vi "Sound Generator Example.vi"() -> ()   [LabVIEW 2018]
uses:
  Waveform Control.xctl
  <vilib>/Waveform/WDTOps.llb/WDT Append Waveforms DBL.vi
panel:
  in  "Show Y=0":bool=TRUE
  in  "Show Scales":bool
  in  "Exit":bool
  in  "Secs to play":dbl=0.25
  in  "Repeats/sec":dbl=478.0
  in  "Play":bool
  in  "Waveform":waveform(dbl)(xcontrol)={"t0"=timestamp(0 s since 1904-01-01), "dt"=0.0, "Y"=[0.0, 0.049067674327418015, 0.0980171403295606, 0.14673047445536175, 0.19509032201612828, 0.2429801799032639, 0.2902846772544624, 0.33688985339222005, 0.3826834323650898, 0.4275550934302821, 0.47139673682599764, 0.5141027441932218, 0.5555702330196022, 0.5956993044924334, 0.6343932841636455, 0.6715589548470184, 0.7071067811865475, 0.7409511253549591, 0.7730104533627369, 0.8032075314806449, 0.8314696123025451, 0.8577286100002721, 0.8819212643483549, 0.9039892931234433, 0.9238795325112866, 0.9415440651830208, 0.9569403357322087, 0.970031253194544, 0.9807852804032303, 0.9891765099647809, 0.9951847266721968, 0.9987954562051723, 0.9999999999999999, 0.9987954562051723, 0.9951847266721968, 0.9891765099647809, 0.9807852804032304, 0.970031253194544, 0.9569403357322088, 0.9415440651830208, 0.9238795325112867, 0.9039892931234433, 0.881921264348355, 0.8577286100002721, 0.8314696123025452, 0.8032075314806449, 0.773010453362737, 0.7409511253549591, 0.7071067811865476, 0.6715589548470184, 0.6343932841636456, 0.5956993044924334, 0.5555702330196023, 0.5141027441932218, 0.4713967368259977, 0.42755509343028214, 0.38268343236508984, 0.3368898533922201, 0.29028467725446244, 0.24298017990326393, 0.19509032201612836, 0.14673047445536178, 0.0980171403295607, 0.04906767432741803, 1.0034968732711147e-16, -0.04906767432741801, -0.0980171403295605, -0.14673047445536175, -0.19509032201612816, -0.2429801799032639, -0.2902846772544623, -0.33688985339222005, -0.38268343236508967, -0.4275550934302821, -0.47139673682599753, -0.5141027441932218, -0.5555702330196021, -0.5956993044924334, -0.6343932841636454, -0.6715589548470184, -0.7071067811865475, -0.7409511253549591, -0.7730104533627369, -0.8032075314806449, -0.8314696123025451, -0.8577286100002721, -0.8819212643483549, -0.9039892931234433, -0.9238795325112866, -0.9415440651830208, -0.9569403357322087, -0.970031253194544, -0.9807852804032303, -0.9891765099647809, -0.9951847266721968, -0.9987954562051723, -0.9999999999999999, -0.9987954562051723, -0.9951847266721968, -0.9891765099647809, -0.9807852804032304, -0.970031253194544, -0.9569403357322088, -0.9415440651830208, -0.9238795325112867, -0.9039892931234433, -0.881921264348355, -0.8577286100002721, -0.8314696123025452, -0.8032075314806449, -0.773010453362737, -0.7409511253549591, -0.7071067811865476, -0.6715589548470184, -0.6343932841636456, -0.5956993044924334, -0.5555702330196023, -0.5141027441932218, -0.4713967368259977, -0.42755509343028214, -0.38268343236508984, -0.3368898533922201, -0.29028467725446244, -0.24298017990326395, -0.19509032201612836, -0.1467304744553618, -0.0980171403295607, -0.049067674327418064], "attributes"=variant("XControl State"=variant(cluster{"Show Axes":bool, "Show Y=0":bool, "Controls":cluster{"Type":enum16{"Level", "Sine", "Triangle", "Ramp", "Saw Tooth", "Square", "Function"}, "Periods":dbl, "Points":i32, "Offset":dbl, "Amplitdue":dbl, "Starting Phase":dbl, "func":string}, "Show Current Location":bool, "Current Location":i32, "dt":dbl, "t0":timestamp} {"Show Axes"=FALSE, "Show Y=0"=TRUE, "Controls"={"Type"=enum."Sine", "Periods"=1.0, "Points"=128, "Offset"=0.0, "Amplitdue"=1.0, "Starting Phase"=0.0, "func"=""}, "Show Current Location"=TRUE, "Current Location"=0, "dt"=0.0, "t0"=timestamp(0 s since 1904-01-01)}))}
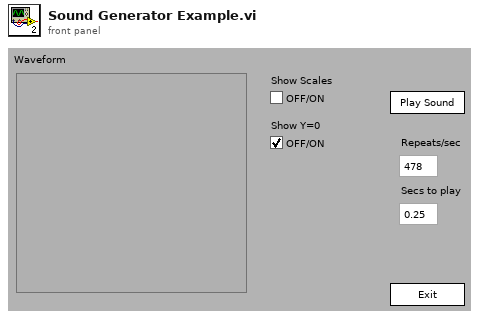
[diagram p1: front panel]
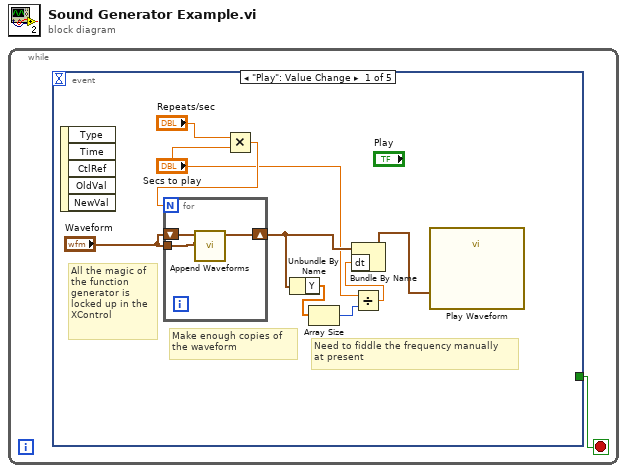
[diagram p0: block diagram]
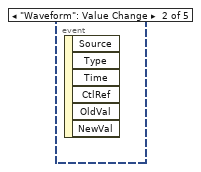
[diagram p2: hidden frame]
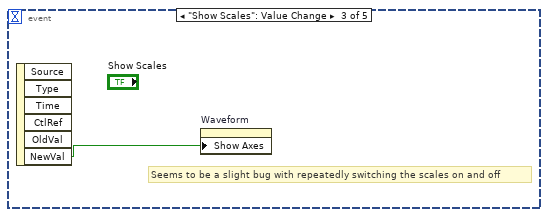
[diagram p3: hidden frame]
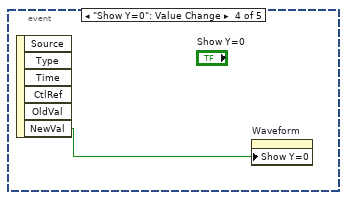
[diagram p4: hidden frame]
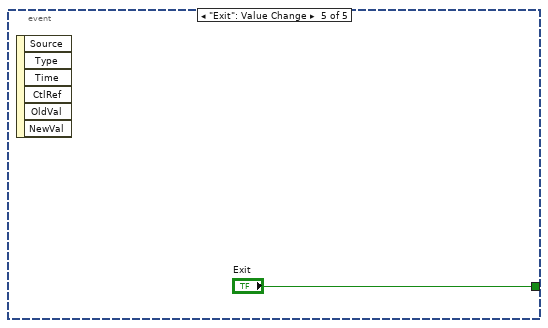
[diagram p5: hidden frame]
diagram:
  n1 = while {
    stop <- w1 stop-if-true
    n2 = event shown="[0] \"Play\": Value Change" {
      selector: _ -> [_ _ _ _ _]
      dyn-events: _ -> [_ _ _ _ _]
      timeout: _ -> [_ _ _ _ _]
      tunnel: [_ _ _ _ "Exit"] -> w1
      event "Play": Value Change {
        # "Need to fiddle the frequency manually\nat present"
        # "Make enough copies of\nthe waveform"
        # "All the magic of\nthe function\ngenerator is\nlocked up in the\nXControl"
        n3 = event-data() -> ()  [unwired: 6 out]
        n4 = Multiply(x="Repeats/sec", y="Secs to play") -> (x*y=w9:dbl)
        n5 = for {
          N: w9 -> [_]
          shift-right: [w13] -> w5
          shift-left: "Waveform" -> [w12]
          tunnel: "Waveform" -> [w11]
          n6 = call-poly <vilib>:"Append Waveforms.vi"("waveform B"=w11, "waveform A"=w12) -> ("waveform out"=w13:waveform(dbl))  [unwired: 1 in, 8 out]
        }
        n7 = Unbundle By Name(w5) -> ("Y"=w7:dbl[])
        n8 = Array Size(array=w7) -> (size(s)=w4:i32)
        n9 = Divide(x="Secs to play", y=w4) -> (x/y=w2:dbl)
        n10 = Bundle By Name(cluster=w5, "dt"=w2) -> (w8:waveform(dbl))
        n11 = call "Play Waveform"("Data"=w8) -> ()  [unwired: 2 in, 17 out]
      }
      event "Waveform": Value Change {
        n12 = event-data() -> ()  [unwired: 7 out]
      }
      event "Show Scales": Value Change {
        # "Seems to be a slight bug with repeatedly switching the scales on and off"
        n13 = event-data() -> ("NewVal"=w14:bool)  [unwired: 6 out]
        n14 = property on="Waveform" class="Waveform Control (strict)"("Show Axes"=w14) -> ()  [unwired: 2 in, 2 out]
      }
      event "Show Y=0": Value Change {
        n15 = event-data() -> ("NewVal"=w15:bool)  [unwired: 6 out]
        n16 = property on="Waveform" class="Waveform Control (strict)"("Show Y=0"=w15) -> ()  [unwired: 2 in, 2 out]
      }
      event "Exit": Value Change {
        n17 = event-data() -> ()  [unwired: 7 out]
      }
    }
  }
